vi "Self correcting directional - ACCEL ver 2.vi"() -> ()   [LabVIEW 2018]
uses:
  <vilib>/Studica/Studica Toolkit/Background/I2C Channel.ctl
  <vilib>/Studica/Studica Toolkit/NavX/NavX.lvlib
  CALIBRATION states.ctl
  Underlying VI's/Elasped Timer/Control.ctl
  <vilib>/Studica/Studica Toolkit/Background/DIO Channel.ctl
panel:
  in  "LED ON":bool
  in  "LED Blink":bool
  in  "stop 2":bool
  in  "Start 2":bool
  out "State 2":T1
  out "Numeric 2":dbl
  out "IN 2":bool
  out "RT Stop 2":bool
  in  "Zero Yaw 2":bool
  out "Yaw 2":dbl
  in  "wTargetSpeed 2":dbl
  in  "yTargetSpeed 2":dbl
  in  "xTargetSpeed 2":dbl
  out "Output\nSpeed 2":T2
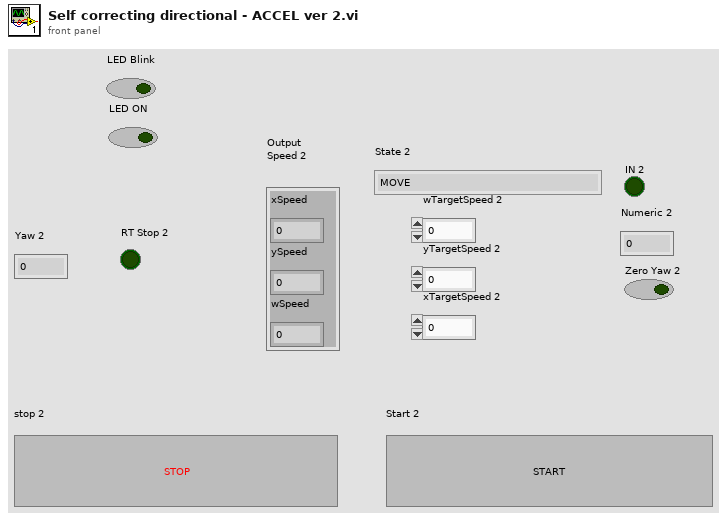
[diagram p1: front panel]
types:
  T1 = typedef "CALIBRATION states.ctl" = enum16{"MOVE", "ACW CALIBRATE", "CW CALIBRATE", "DIR CHECK", "IDLE", "INIT"}
  T2 = cluster{"xSpeed":dbl, "ySpeed":dbl, "wSpeed":dbl}
  T3 = typedef "DIO Channel.ctl" = enum16{"Not Connected", "A/DIO1", "A/DIO2", "A/DIO3", "A/DIO4", "A/DIO5", "A/DIO6", "A/DIO7", "A/DIO13", "B/DIO1", "B/DIO2", "B/DIO3", "B/DIO4", "B/DIO5", "B/DIO6", "B/DIO7", "B/DIO13", "C/DIO0", "C/DIO1", "C/DIO2", "C/DIO3", "C/DIO4", "C/DIO5", "C/DIO6", "C/DIO7"}
  T4 = typedef "I2C Channel.ctl" = enum16{"Not Connected", "A", "B"}
  T5 = typedef "Control.ctl" = enum16{"Start", "Pause", "Initialize"}
  T6 = cluster{"DIO Channel":T3, "FPGA VI Reference Out":refnum<k20>}
  T7 = cluster{"I2C Ref Out":cluster{"I2C Channel":T4, "FPGA VI Reference Out":refnum<k20>}, "Connected":bool, "Slave Address (7-bit)":u8, "Registry":u8[]}
  T8 = cluster{"Yaw":dbl, "Roll":dbl, "Pitch":dbl, "Heading":dbl, "Fused Heading":dbl}
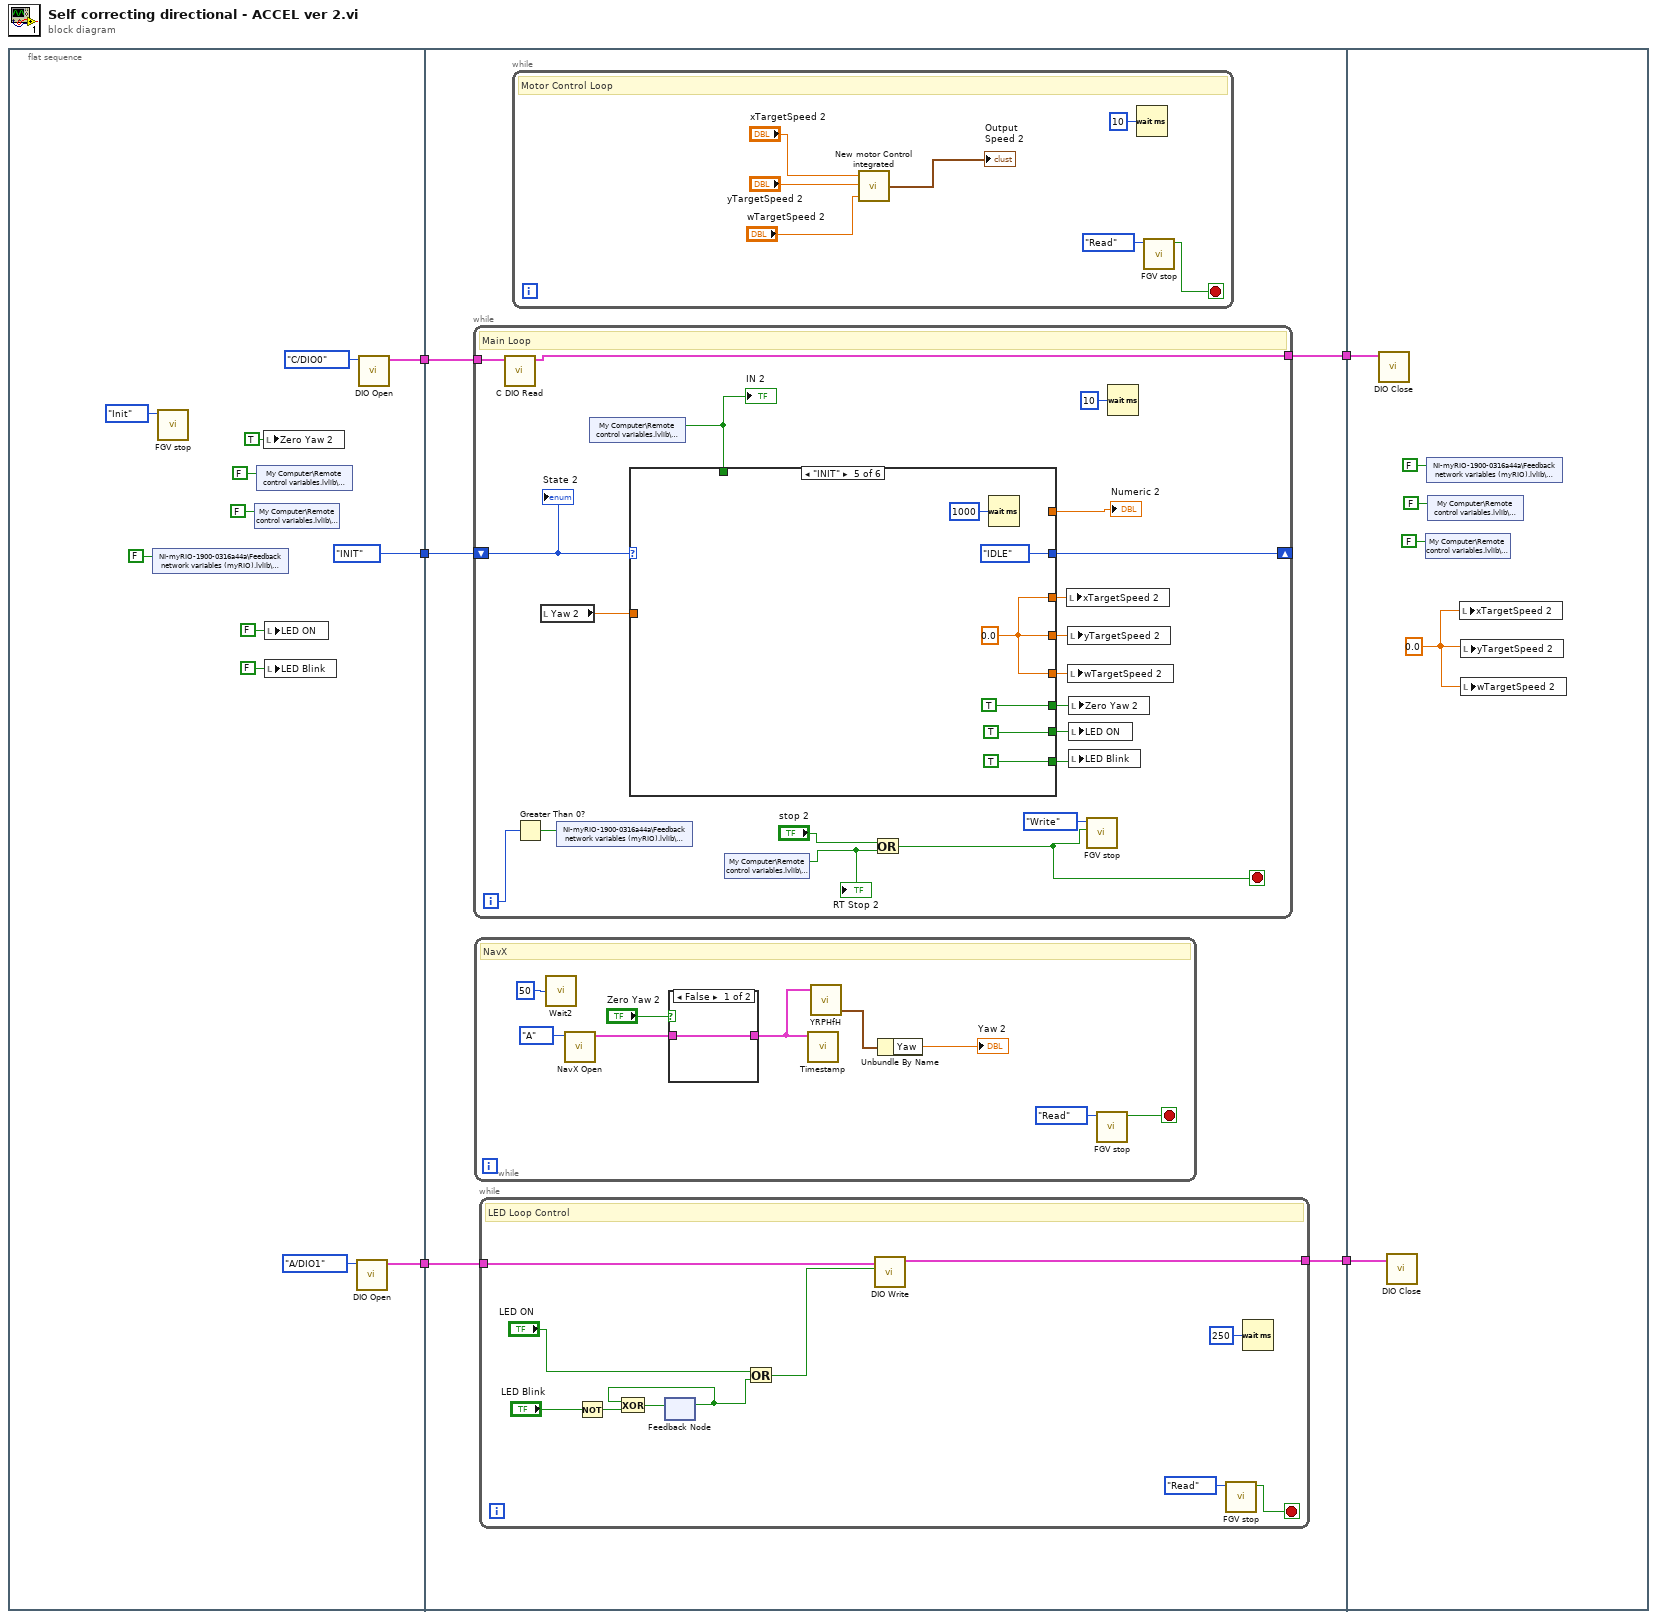
[diagram p0: block diagram]
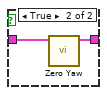
[diagram p2: hidden frame]
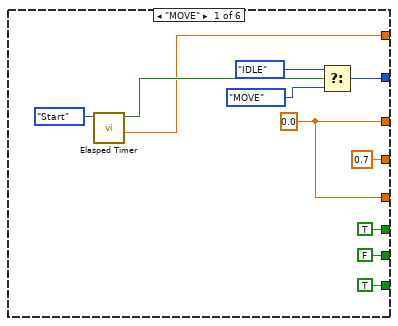
[diagram p3: hidden frame]
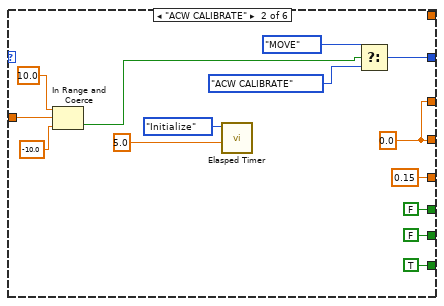
[diagram p4: hidden frame]
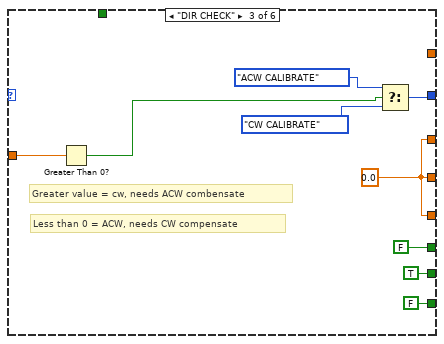
[diagram p5: hidden frame]
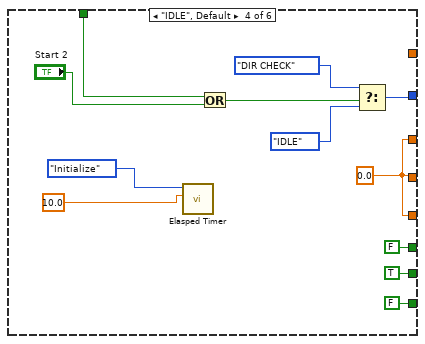
[diagram p6: hidden frame]
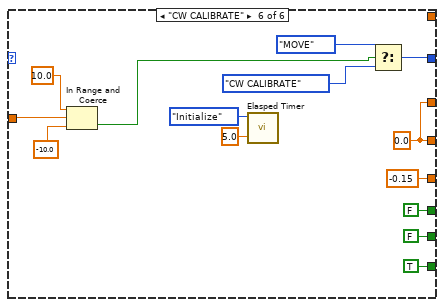
[diagram p7: hidden frame]
diagram:
  n1 = flat-sequence {
    tunnel: [CALIBRATION_states."INIT"] -> w5
    tunnel: [w13] -> w4
    tunnel: [w8] -> w2
    tunnel: w5 -> [w22]
    tunnel: w4 -> [w21]
    tunnel: [w20] -> w3
    tunnel: w2 -> [w19]
    tunnel: [w18] -> w1
    tunnel: w3 -> [w143]
    tunnel: w1 -> [w140]
    frame #0 {
      n2 = shared-variable "NI-myRIO-1900-0316a44a\\Feedback network variables (myRIO).lvlib\\Program running"(FALSE ("Program running")) -> ()  [unwired: 1 in, 1 out]
      n3 = call "FGV stop.vi"("States"=enum16{"Read", "Write", "Init"}."Init") -> ()  [unwired: 9 in, 2 out]
      n4 = shared-variable "My Computer\\Remote control variables.lvlib\\RT Stop"(FALSE ("RT Stop")) -> ()  [unwired: 1 in, 1 out]
      n5 = shared-variable "My Computer\\Remote control variables.lvlib\\ServoGrip"(FALSE ("ServoGrip")) -> ()  [unwired: 1 in, 1 out]
      n6 = local write "Zero Yaw 2"(TRUE ("Zero Yaw")) -> ()
      n7 = local write "LED ON"(FALSE ("LED ON")) -> ()
      n8 = local write "LED Blink"(FALSE ("LED Blink")) -> ()
      n9 = call <vilib>:"DIO Open.vi"("DIO Channel"=DIO_Channel."A/DIO1") -> ("DIO Info Out"=w8:T6)  [unwired: 9 in, 1 out]
      n10 = call <vilib>:"DIO Open.vi"("DIO Channel"=DIO_Channel."C/DIO0") -> ("DIO Info Out"=w13:T6)  [unwired: 9 in, 1 out]
    }
    frame #1 {
      n11 = while {
        shift-right: [w64] -> _
        shift-left: w22 -> [w70]
        tunnel: w21 -> [w62]
        tunnel: [w61] -> w20
        i -> [w54]
        stop <- w58 stop-if-true
        # "Main Loop"
        n12 = call <vilib>:"C DIO Read.vi"("DIO Info In in"=w62) -> ("DIO Info In out"=w61:T6)  [unwired: 8 in, 2 out]
        n13 = Greater Than 0?(x=w54) -> (x > 0?=w53:bool)
        n14 = local read "Yaw 2"() -> (w69:dbl)
        n15 = shared-variable "NI-myRIO-1900-0316a44a\\Feedback network variables (myRIO).lvlib\\Program running"(w53) -> ()  [unwired: 1 in, 1 out]
        n16 = shared-variable "My Computer\\Remote control variables.lvlib\\ServoGrip"() -> (w57:bool)  [unwired: 1 in, 1 out]
        "IN 2" <- w57
        n17 = case shown="\"INIT\"" w70 {
          tunnel: w69 -> [_ w94 w103 _ _ w130]
          tunnel: [0.7 w88 w101 w115 w124 w129] -> w68
          tunnel: [w77 w88 w101 w115 w124 w129] -> w67
          tunnel: [w77 0.15 w101 w115 w124 -0.15] -> w66
          tunnel: [TRUE FALSE FALSE FALSE TRUE FALSE] -> w65
          tunnel: [w83 w97 w106 w118 CALIBRATION_states."IDLE" w131] -> w64
          tunnel: [w75 _ _ _ _ _] -> w63
          tunnel: w57 -> [_ _ _ w109 _ _]
          tunnel: [FALSE FALSE TRUE TRUE TRUE FALSE] -> w56
          tunnel: [TRUE TRUE FALSE FALSE TRUE TRUE] -> w55
          frame "MOVE" {
            w77 = 0.0
            n18 = call "Elasped Timer.vi"("Action"=Control."Start") -> ("Elapsed Time"=w75:dbl, "Time Out?!"=w79:bool)  [unwired: 7 in, 2 out]
            n19 = Select(t=CALIBRATION_states."IDLE", s=w79, f=CALIBRATION_states."MOVE") -> (s? t:f=w83:T1)
          }
          frame "ACW CALIBRATE" {
            w88 = 0.0
            n20 = In Range and Coerce(upper limit=10.0, x=w94, lower limit=-10.0) -> (In Range?=w91:bool)  [unwired: 1 out]
            n21 = call "Elasped Timer.vi"("Time Setting"=5.0, "Action"=Control."Initialize") -> ()  [unwired: 6 in, 4 out]
            n22 = Select(t=CALIBRATION_states."MOVE", s=w91, f=CALIBRATION_states."ACW CALIBRATE") -> (s? t:f=w97:T1)
          }
          frame "DIR CHECK" {
            w101 = 0.0
            # "Less than 0 = ACW, needs CW compensate"
            # "Greater value = cw, needs ACW combensate"
            n23 = Greater Than 0?(x=w103) -> (x > 0?=w102:bool)
            n24 = Select(t=CALIBRATION_states."ACW CALIBRATE", s=w102, f=CALIBRATION_states."CW CALIBRATE") -> (s? t:f=w106:T1)
          }
          frame "IDLE", Default {
            w115 = 0.0
            n25 = call "Elasped Timer.vi"("Time Setting"=10.0, "Action"=Control."Initialize") -> ()  [unwired: 6 in, 4 out]
            n26 = Or(x=w109, y="Start 2") -> (x .or. y?=w110:bool)
            n27 = Select(t=CALIBRATION_states."DIR CHECK", s=w110, f=CALIBRATION_states."IDLE") -> (s? t:f=w118:T1)
          }
          frame "INIT" {
            w124 = 0.0
            n28 = Wait (ms)(milliseconds to wait=u32 1000) -> ()  [unwired: 1 out]
          }
          frame "CW CALIBRATE" {
            w129 = 0.0
            n29 = In Range and Coerce(upper limit=10.0, x=w130, lower limit=-10.0) -> (In Range?=w136:bool)  [unwired: 1 out]
            n30 = call "Elasped Timer.vi"("Time Setting"=5.0, "Action"=Control."Initialize") -> ()  [unwired: 6 in, 4 out]
            n31 = Select(t=CALIBRATION_states."MOVE", s=w136, f=CALIBRATION_states."CW CALIBRATE") -> (s? t:f=w131:T1)
          }
        }
        "Numeric 2" <- w63
        n32 = shared-variable "My Computer\\Remote control variables.lvlib\\RT Stop"() -> (w59:bool)  [unwired: 1 in, 1 out]
        "RT Stop 2" <- w59
        n33 = Or(x="stop 2", y=w59) -> (x .or. y?=w58:bool)
        n34 = local write "xTargetSpeed 2"(w67) -> ()
        n35 = local write "yTargetSpeed 2"(w68) -> ()
        n36 = local write "wTargetSpeed 2"(w66) -> ()
        n37 = local write "Zero Yaw 2"(w65) -> ()
        n38 = local write "LED ON"(w56) -> ()
        n39 = local write "LED Blink"(w55) -> ()
        n40 = call "FGV stop.vi"("Stop Input"=w58, "States"=enum16{"Read", "Write", "Init"}."Write") -> ()  [unwired: 8 in, 2 out]
        n41 = Wait (ms)(milliseconds to wait=u32 10) -> ()  [unwired: 1 out]
        "State 2" <- w70
      }
      n42 = while {
        stop <- w44 stop-if-true
        # "NavX"
        n43 = call "Wait2"("Count(mSec)"=u32 50) -> ()  [unwired: 1 out]
        n44 = call <vilib>:"NavX Open.vi"("I2C Channel"=I2C_Channel."A") -> ("NavX Info"=w48:T7)  [unwired: 9 in, 1 out]
        n45 = case shown="False" "Zero Yaw 2" {
          tunnel: w48 -> [w50 w52]
          tunnel: [w50 w51] -> w49
          frame False {
          }
          frame True {
            n46 = call <vilib>:"Zero Yaw.vi"("NavX Info In"=w52) -> ("NavX Info Out"=w51:T7)  [unwired: 10 in]
          }
        }
        n47 = call <vilib>:"Timestamp.vi"("NavX Info In"=w49) -> ()  [unwired: 9 in, 2 out]
        n48 = call <vilib>:"YRPHfH.vi"("NavX Info In"=w49) -> ("YRPHfH"=w42:T8)  [unwired: 3 in, 1 out]
        n49 = Unbundle By Name(w42) -> ("Yaw"=→"Yaw 2":dbl)
        n50 = call "FGV stop.vi"("States"=enum16{"Read", "Write", "Init"}."Read") -> ("stop Output"=w44:bool)  [unwired: 9 in, 1 out]
      }
      n51 = while {
        tunnel: w19 -> [w25]
        tunnel: [w24] -> w18
        stop <- w27 stop-if-true
        # "LED Loop Control"
        n52 = Not(x="LED Blink") -> (.not. x?=w32:bool)
        n53 = feedback #1() -> (w29:bool)  [unwired: 1 in]
        n54 = Exclusive Or(1:w32, 2:w29) -> (0:w33:bool)
        n55 = feedback-in #1(w33) -> ()
        n56 = Or(x="LED ON", y=w29) -> (x .or. y?=w23:bool)
        n57 = call <vilib>:"DIO Write.vi"("Input"=w23, "DIO Info In"=w25) -> ("DIO Info Out"=w24:T6)  [unwired: 8 in, 1 out]
        n58 = call "FGV stop.vi"("States"=enum16{"Read", "Write", "Init"}."Read") -> ("stop Output"=w27:bool)  [unwired: 9 in, 1 out]
        n59 = Wait (ms)(milliseconds to wait=u32 250) -> ()  [unwired: 1 out]
      }
      n60 = while {
        stop <- w40 stop-if-true
        # "Motor Control Loop"
        n61 = call "New motor Control integrated.vi"("wTargetSpeed"="wTargetSpeed 2", "yTargetSpeed"="yTargetSpeed 2", "xTargetSpeed"="xTargetSpeed 2") -> ("Speed"=→"Output\nSpeed 2":T2)
        n62 = Wait (ms)(milliseconds to wait=u32 10) -> ()  [unwired: 1 out]
        n63 = call "FGV stop.vi"("States"=enum16{"Read", "Write", "Init"}."Read") -> ("stop Output"=w40:bool)  [unwired: 9 in, 1 out]
      }
    }
    frame #2 {
      w144 = 0.0
      n64 = call <vilib>:"DIO Close.vi"("DIO Info In"=w143) -> ()  [unwired: 10 in, 1 out]
      n65 = call <vilib>:"DIO Close.vi"("DIO Info In"=w140) -> ()  [unwired: 10 in, 1 out]
      n66 = shared-variable "My Computer\\Remote control variables.lvlib\\RT Stop"(FALSE ("RT Stop")) -> ()  [unwired: 1 in, 1 out]
      n67 = shared-variable "NI-myRIO-1900-0316a44a\\Feedback network variables (myRIO).lvlib\\Program running"(FALSE ("Program running")) -> ()  [unwired: 1 in, 1 out]
      n68 = shared-variable "My Computer\\Remote control variables.lvlib\\ServoGrip"(FALSE ("ServoGrip")) -> ()  [unwired: 1 in, 1 out]
      n69 = local write "xTargetSpeed 2"(w144) -> ()
      n70 = local write "yTargetSpeed 2"(w144) -> ()
      n71 = local write "wTargetSpeed 2"(w144) -> ()
    }
  }
